vi "setMaxSpeed_DriveQuadTalonSRX.vi"(10 "MAX DESIRED\nVELOCITY (UNITS)":dbl=10.0 format="%.4f") -> (1 "1 / Max Speed":dbl format="%.4f", 3 "Max Speed":dbl format="%.4f")   [LabVIEW 2019, in "DriveQuadTalonSRX_Motor.lvlib"]
uses:
  DriveQuadTalonSRX_Motor.lvlib
  globals_DriveQuadTalonSRX.vi
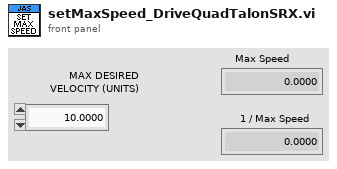
[diagram p1: front panel]
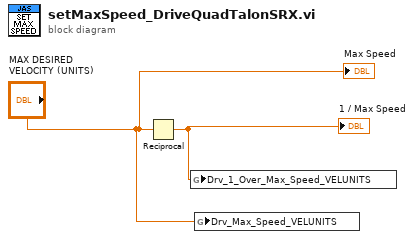
[diagram p0: block diagram]
diagram:
  n1 = Reciprocal(x="MAX DESIRED\nVELOCITY (UNITS)") -> (1/x=w2:dbl)
  "1 / Max Speed" <- w2
  n2 = global write "globals_DriveQuadTalonSRX.vi" "Drv_1_Over_Max_Speed_VELUNITS"(w2) -> ()
  n3 = global write "globals_DriveQuadTalonSRX.vi" "Drv_Max_Speed_VELUNITS"("MAX DESIRED\nVELOCITY (UNITS)") -> ()
  "Max Speed" <- "MAX DESIRED\nVELOCITY (UNITS)"
